vi "Create Axis Captions.vi"(6 "Label Width":sgl, 7 "Which Axis?":T1(ring)=enum."Z Opposite", 8 "error in (no error)":errorcluster, 9 "Caption Size":u16, 10 "Caption Color":u32(colorbox), 11 "Caption Text":string) -> (0 "error out":errorcluster, 3 "New Caption Object":refnum<vi>)   [LabVIEW 2020, in "3D Plot.lvclass"]
uses:
  3D Plot.lvclass
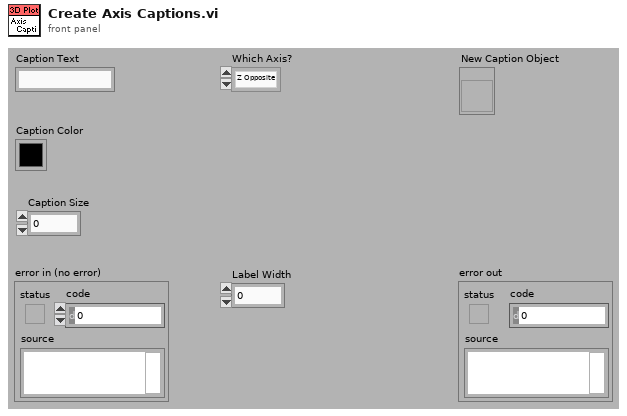
[diagram p1: front panel]
types:
  T1 = enum16{"X", "Y", "Z", "X Opposite", "Y Opposite", "Z Opposite"}
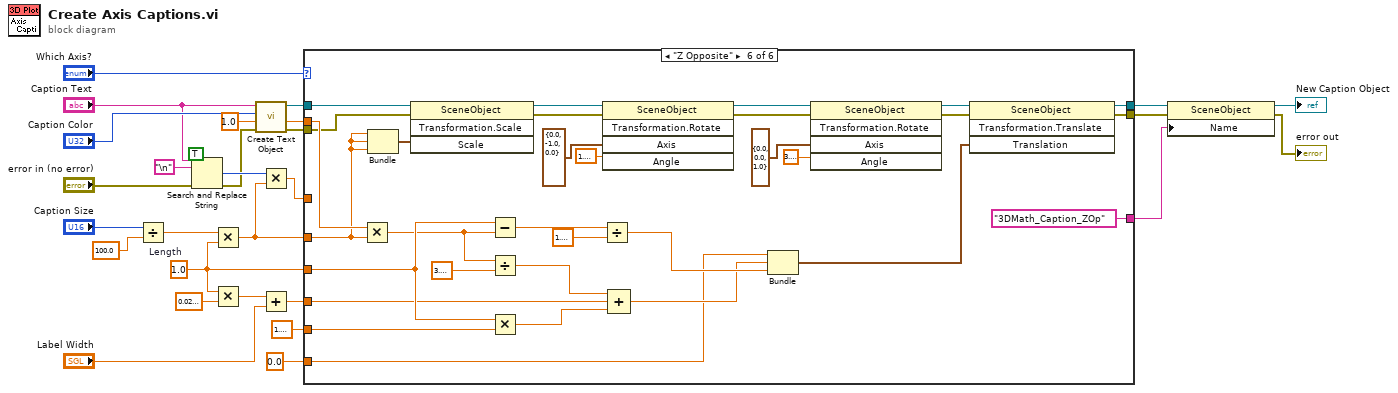
[diagram p0: block diagram]
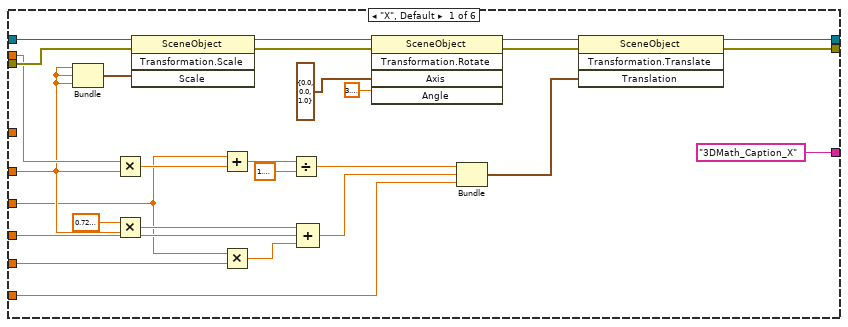
[diagram p2: hidden frame]
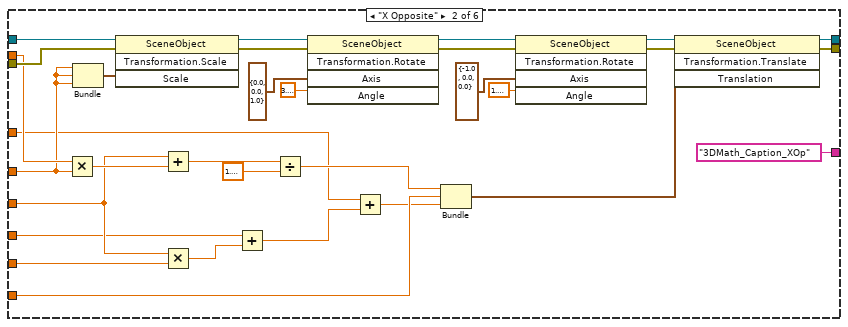
[diagram p3: hidden frame]
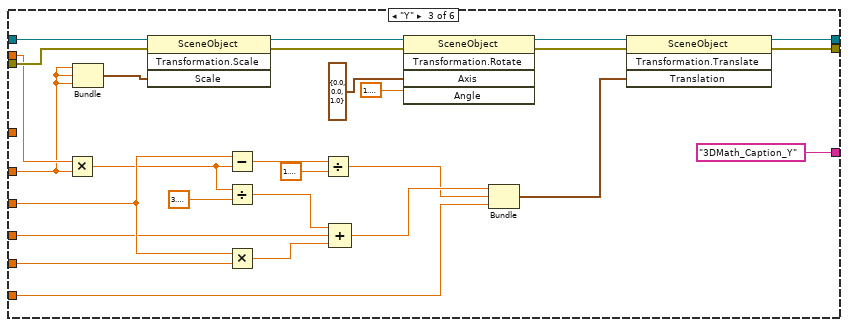
[diagram p4: hidden frame]
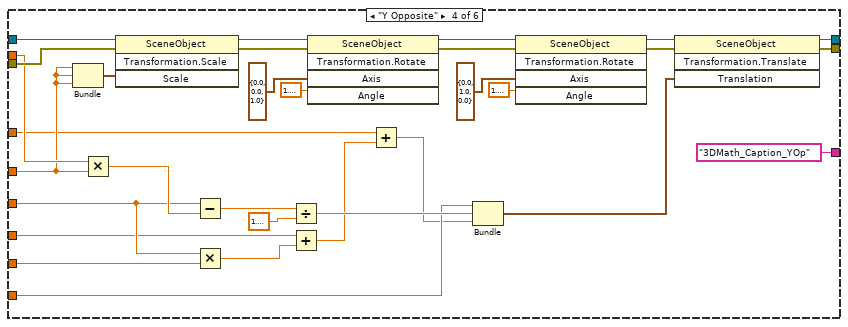
[diagram p5: hidden frame]
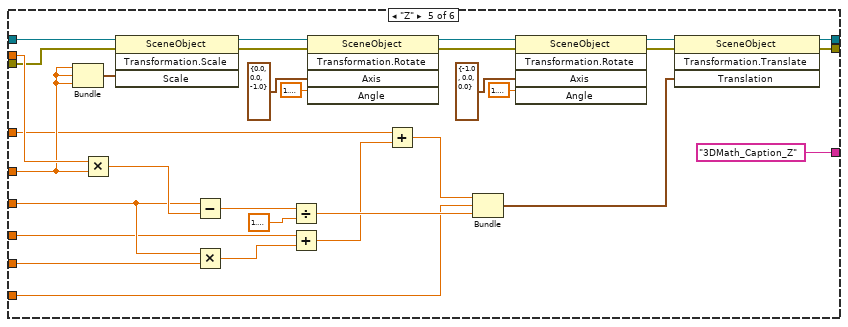
[diagram p6: hidden frame]
diagram:
  w1 = sgl 1.0  # Length
  n1 = Divide(x="Caption Size", y=sgl 100.0 ("x")) -> (x/y=w4:sgl)
  n2 = Search and Replace String(replace all?=TRUE ("replace all? (F)"), input string="Caption Text", search string="\n", error in="error in (no error)") -> (number of replacements=w16:i32, error out=w14:errorcluster)  [unwired: 4 in, 2 out]
  n3 = Multiply(x=w4, y=w1) -> (x*y=w2:sgl)
  n4 = Multiply(x=w1, y=sgl 0.03) -> (x*y=w7:sgl)
  n5 = call "Create Text Object.vi"("error in (no error)"=w14, "Alpha"=sgl 1.0, "Color Box"="Caption Color", "Value String"="Caption Text") -> ("error out"=w23:errorcluster, "Numeric"=w22:sgl, "Scene:New Object"=w21:refnum<vi>)  [unwired: 5 out]
  n6 = Multiply(x=w16, y=w2) -> (x*y=w18:sgl)
  n7 = Add(x=w7, y="Label Width") -> (x+y=w5:sgl)
  n8 = case shown="\"Z Opposite\"" "Which Axis?" {
    tunnel: w23 -> [w56 w69 w102 w128 w157 w190]
    tunnel: w22 -> [w55 w68 w101 w127 w158 w191]
    tunnel: w21 -> [w54 w70 w103 w129 w159 w192]
    tunnel: [w53 w64 w99 w122 w152 w186] -> w11
    tunnel: [w50 w63 w100 w123 w153 w187] -> w27
    tunnel: w1 -> [w35 w66 w97 w125 w155 w188]
    tunnel: w5 -> [w49 w65 w92 w124 w154 w182]
    tunnel: w2 -> [w48 w67 w98 w126 w156 w189]
    tunnel: sgl 1.1 ("y") -> [w34 w62 w91 w121 w151 w180]
    tunnel: sgl 0.0 ("x+y") -> [w32 w61 w90 w118 w150 w179]
    tunnel: w18 -> [_ w59 _ w120 w149 _]
    tunnel: ["3DMath_Caption_X" "3DMath_Caption_XOp" "3DMath_Caption_Y" "3DMath_Caption_YOp" "3DMath_Caption_Z" "3DMath_Caption_ZOp"] -> w10
    frame "X", Default {
      n9 = Bundle(w48, w48, w48) -> (w38:cluster{sgl, sgl, sgl})  [unwired: 1 out]
      n10 = Multiply(x=w55, y=w48) -> (x*y=w44:sgl)
      n11 = Multiply(x=sgl 0.72, y=w48) -> (x*y=w37:sgl)
      n12 = invoke class="SceneObject" method="Transformation.Scale"(reference=w54, error in=w56, "Scale"=w38) -> (reference out=w40:refnum<vi>, error out=w51:errorcluster)  [unwired: 1 in, 2 out]
      n13 = Add(x=w35, y=w44) -> (x+y=w45:sgl)
      n14 = Multiply(x=w35, y=w34) -> (x*y=w33:sgl)
      n15 = Divide(x=w45, y=sgl 1.9) -> (x/y=w47:sgl)
      n16 = Compound Arithmetic op=ADD(w37, w49, w33) -> (w31:sgl)
      n17 = invoke class="SceneObject" method="Transformation.Rotate"(reference=w40, error in=w51, "Axis"=cluster{"X":sgl, "Y":sgl, "Z":sgl} {"X"=0.0, "Y"=0.0, "Z"=1.0}, "Angle"=sgl 3.1415927) -> (reference out=w39:refnum<vi>, error out=w52:errorcluster)  [unwired: 1 in, 3 out]
      n18 = Bundle(w47, w31, "x+y"=w32) -> (w43:cluster{sgl, sgl, "x+y":sgl})  [unwired: 1 out]
      n19 = invoke class="SceneObject" method="Transformation.Translate"(reference=w39, error in=w52, "Translation"=w43) -> (reference out=w50:refnum<vi>, error out=w53:errorcluster)  [unwired: 1 in, 2 out]
    }
    frame "X Opposite" {
      n20 = Multiply(x=w68, y=w67) -> (x*y=w86:sgl)
      n21 = Bundle(w67, w67, w67) -> (w74:cluster{sgl, sgl, sgl})  [unwired: 1 out]
      n22 = invoke class="SceneObject" method="Transformation.Scale"(reference=w70, error in=w69, "Scale"=w74) -> (reference out=w87:refnum<vi>, error out=w73:errorcluster)  [unwired: 1 in, 2 out]
      n23 = Add(x=w66, y=w86) -> (x+y=w85:sgl)
      n24 = Multiply(x=w66, y=w62) -> (x*y=w83:sgl)
      n25 = Add(x=w65, y=w83) -> (x+y=w60:sgl)
      n26 = Divide(x=w85, y=sgl 1.9) -> (x/y=w75:sgl)
      n27 = invoke class="SceneObject" method="Transformation.Rotate"(reference=w87, error in=w73, "Axis"=cluster{"X":sgl, "Y":sgl, "Z":sgl} {"X"=0.0, "Y"=0.0, "Z"=1.0}, "Angle"=sgl 3.1415927) -> (reference out=w82:refnum<vi>, error out=w72:errorcluster)  [unwired: 1 in, 3 out]
      n28 = Add(x=w59, y=w60) -> (x+y=w58:sgl)
      n29 = Bundle(w75, "x+y"=w61, w58) -> (w81:cluster{sgl, "x+y":sgl, sgl})  [unwired: 1 out]
      n30 = invoke class="SceneObject" method="Transformation.Rotate"(reference=w82, error in=w72, "Axis"=cluster{"X":sgl, "Y":sgl, "Z":sgl} {"X"=-1.0, "Y"=0.0, "Z"=0.0}, "Angle"=sgl 1.5707964) -> (reference out=w76:refnum<vi>, error out=w71:errorcluster)  [unwired: 1 in, 3 out]
      n31 = invoke class="SceneObject" method="Transformation.Translate"(reference=w76, error in=w71, "Translation"=w81) -> (reference out=w63:refnum<vi>, error out=w64:errorcluster)  [unwired: 1 in, 2 out]
    }
    frame "Y" {
      n32 = Multiply(x=w101, y=w98) -> (x*y=w94:sgl)
      n33 = Bundle(w98, w98, w98) -> (w104:cluster{sgl, sgl, sgl})  [unwired: 1 out]
      n34 = invoke class="SceneObject" method="Transformation.Scale"(reference=w103, error in=w102, "Scale"=w104) -> (reference out=w111:refnum<vi>, error out=w113:errorcluster)  [unwired: 1 in, 2 out]
      n35 = Subtract(x=w97, y=w94) -> (x-y=w105:sgl)
      n36 = Divide(x=w94, y=sgl 3.7) -> (x/y=w95:sgl)
      n37 = Multiply(x=w97, y=w91) -> (x*y=w89:sgl)
      n38 = Divide(x=w105, y=sgl 1.8) -> (x/y=w96:sgl)
      n39 = Compound Arithmetic op=ADD(w95, w92, w89) -> (w112:sgl)
      n40 = invoke class="SceneObject" method="Transformation.Rotate"(reference=w111, error in=w113, "Axis"=cluster{"X":sgl, "Y":sgl, "Z":sgl} {"X"=0.0, "Y"=0.0, "Z"=1.0}, "Angle"=sgl 1.5707964) -> (reference out=w110:refnum<vi>, error out=w114:errorcluster)  [unwired: 1 in, 3 out]
      n41 = Bundle(w112, w96, "x+y"=w90) -> (w107:cluster{sgl, sgl, "x+y":sgl})  [unwired: 1 out]
      n42 = invoke class="SceneObject" method="Transformation.Translate"(reference=w110, error in=w114, "Translation"=w107) -> (reference out=w100:refnum<vi>, error out=w99:errorcluster)  [unwired: 1 in, 2 out]
    }
    frame "Y Opposite" {
      n43 = Bundle(w126, w126, w126) -> (w130:cluster{sgl, sgl, sgl})  [unwired: 1 out]
      n44 = Multiply(x=w127, y=w126) -> (x*y=w132:sgl)
      n45 = invoke class="SceneObject" method="Transformation.Scale"(reference=w129, error in=w128, "Scale"=w130) -> (reference out=w131:refnum<vi>, error out=w143:errorcluster)  [unwired: 1 in, 2 out]
      n46 = Subtract(x=w125, y=w132) -> (x-y=w133:sgl)
      n47 = Multiply(x=w125, y=w121) -> (x*y=w135:sgl)
      n48 = Divide(x=w133, y=sgl 1.8) -> (x/y=w119:sgl)
      n49 = Add(x=w124, y=w135) -> (x+y=w117:sgl)
      n50 = invoke class="SceneObject" method="Transformation.Rotate"(reference=w131, error in=w143, "Axis"=cluster{"X":sgl, "Y":sgl, "Z":sgl} {"X"=0.0, "Y"=0.0, "Z"=1.0}, "Angle"=sgl 1.5707964) -> (reference out=w136:refnum<vi>, error out=w144:errorcluster)  [unwired: 1 in, 3 out]
      n51 = Add(x=w120, y=w117) -> (x+y=w116:sgl)
      n52 = Bundle("x+y"=w118, w119, w116) -> (w137:cluster{"x+y":sgl, sgl, sgl})  [unwired: 1 out]
      n53 = invoke class="SceneObject" method="Transformation.Rotate"(reference=w136, error in=w144, "Axis"=cluster{"X":sgl, "Y":sgl, "Z":sgl} {"X"=0.0, "Y"=1.0, "Z"=0.0}, "Angle"=sgl 1.5707964) -> (reference out=w141:refnum<vi>, error out=w145:errorcluster)  [unwired: 1 in, 3 out]
      n54 = invoke class="SceneObject" method="Transformation.Translate"(reference=w141, error in=w145, "Translation"=w137) -> (reference out=w123:refnum<vi>, error out=w122:errorcluster)  [unwired: 1 in, 2 out]
    }
    frame "Z" {
      n55 = Bundle(w156, w156, w156) -> (w160:cluster{sgl, sgl, sgl})  [unwired: 1 out]
      n56 = Multiply(x=w158, y=w156) -> (x*y=w162:sgl)
      n57 = invoke class="SceneObject" method="Transformation.Scale"(reference=w159, error in=w157, "Scale"=w160) -> (reference out=w161:refnum<vi>, error out=w174:errorcluster)  [unwired: 1 in, 2 out]
      n58 = Subtract(x=w155, y=w162) -> (x-y=w163:sgl)
      n59 = Multiply(x=w155, y=w151) -> (x*y=w165:sgl)
      n60 = Divide(x=w163, y=sgl 1.8) -> (x/y=w173:sgl)
      n61 = Add(x=w154, y=w165) -> (x+y=w148:sgl)
      n62 = invoke class="SceneObject" method="Transformation.Rotate"(reference=w161, error in=w174, "Axis"=cluster{"X":sgl, "Y":sgl, "Z":sgl} {"X"=0.0, "Y"=0.0, "Z"=-1.0}, "Angle"=sgl 1.5707964) -> (reference out=w166:refnum<vi>, error out=w175:errorcluster)  [unwired: 1 in, 3 out]
      n63 = Add(x=w149, y=w148) -> (x+y=w147:sgl)
      n64 = Bundle(w147, "x+y"=w150, w173) -> (w167:cluster{sgl, "x+y":sgl, sgl})  [unwired: 1 out]
      n65 = invoke class="SceneObject" method="Transformation.Rotate"(reference=w166, error in=w175, "Axis"=cluster{"X":sgl, "Y":sgl, "Z":sgl} {"X"=-1.0, "Y"=0.0, "Z"=0.0}, "Angle"=sgl 1.5707964) -> (reference out=w171:refnum<vi>, error out=w176:errorcluster)  [unwired: 1 in, 3 out]
      n66 = invoke class="SceneObject" method="Transformation.Translate"(reference=w171, error in=w176, "Translation"=w167) -> (reference out=w153:refnum<vi>, error out=w152:errorcluster)  [unwired: 1 in, 2 out]
    }
    frame "Z Opposite" {
      n67 = Multiply(x=w191, y=w189) -> (x*y=w183:sgl)
      n68 = Bundle(w189, w189, w189) -> (w207:cluster{sgl, sgl, sgl})  [unwired: 1 out]
      n69 = invoke class="SceneObject" method="Transformation.Scale"(reference=w192, error in=w190, "Scale"=w207) -> (reference out=w206:refnum<vi>, error out=w195:errorcluster)  [unwired: 1 in, 2 out]
      n70 = Subtract(x=w188, y=w183) -> (x-y=w205:sgl)
      n71 = Divide(x=w183, y=sgl 3.7) -> (x/y=w184:sgl)
      n72 = Multiply(x=w188, y=w180) -> (x*y=w178:sgl)
      n73 = Divide(x=w205, y=sgl 1.8) -> (x/y=w201:sgl)
      n74 = invoke class="SceneObject" method="Transformation.Rotate"(reference=w206, error in=w195, "Axis"=cluster{"X":dbl, "Y":dbl, "Z":dbl} {"X"=0.0, "Y"=-1.0, "Z"=0.0}, "Angle"=sgl 1.5707964) -> (reference out=w198:refnum<vi>, error out=w194:errorcluster)  [unwired: 1 in, 3 out]
      n75 = Compound Arithmetic op=ADD(w184, w182, w178) -> (w181:sgl)
      n76 = Bundle("x+y"=w179, w181, w201) -> (w203:cluster{"x+y":sgl, sgl, sgl})  [unwired: 1 out]
      n77 = invoke class="SceneObject" method="Transformation.Rotate"(reference=w198, error in=w194, "Axis"=cluster{"X":dbl, "Y":dbl, "Z":dbl} {"X"=0.0, "Y"=0.0, "Z"=1.0}, "Angle"=sgl 3.1415927) -> (reference out=w197:refnum<vi>, error out=w193:errorcluster)  [unwired: 1 in, 3 out]
      n78 = invoke class="SceneObject" method="Transformation.Translate"(reference=w197, error in=w193, "Translation"=w203) -> (reference out=w187:refnum<vi>, error out=w186:errorcluster)  [unwired: 1 in, 2 out]
    }
  }
  n79 = property class="SceneObject"(reference=w27, error in=w11, "Name"=w10) -> (reference out=→"New Caption Object":refnum<vi>, error out=→"error out":errorcluster)
